vi "Test10.vi"(5 "Peak":T2=enum."PCAN_USBBUS1", 7 "L2T":T1 caption="Limites de test pris en compte", 8 "errin":errorcluster, 9 "SN":string="0B5MEVA000CA1JC1M0000041", 10 "OCV":string) -> (0 "errout":errorcluster, 2 "chaîne concaténée":string, 4 "cluster de sortie":T3, 6 "v1":string)   [LabVIEW 2020]
uses:
  <userlib>/PCAN Basic/Controls/Channel.ctl
  Ctrl/L2T.ctl
  VarGLO/Global var.vi
  <vilib>/regexp/Match Regular Expression.xnode
  <userlib>/PCAN Basic/PCANBasic.lvlib
panel:
  out "String out":string
  # "Pre DCIR_____________________________________"
  # "intra DCIR_____________________________________"
  # "Post DCIR_____________________________________"
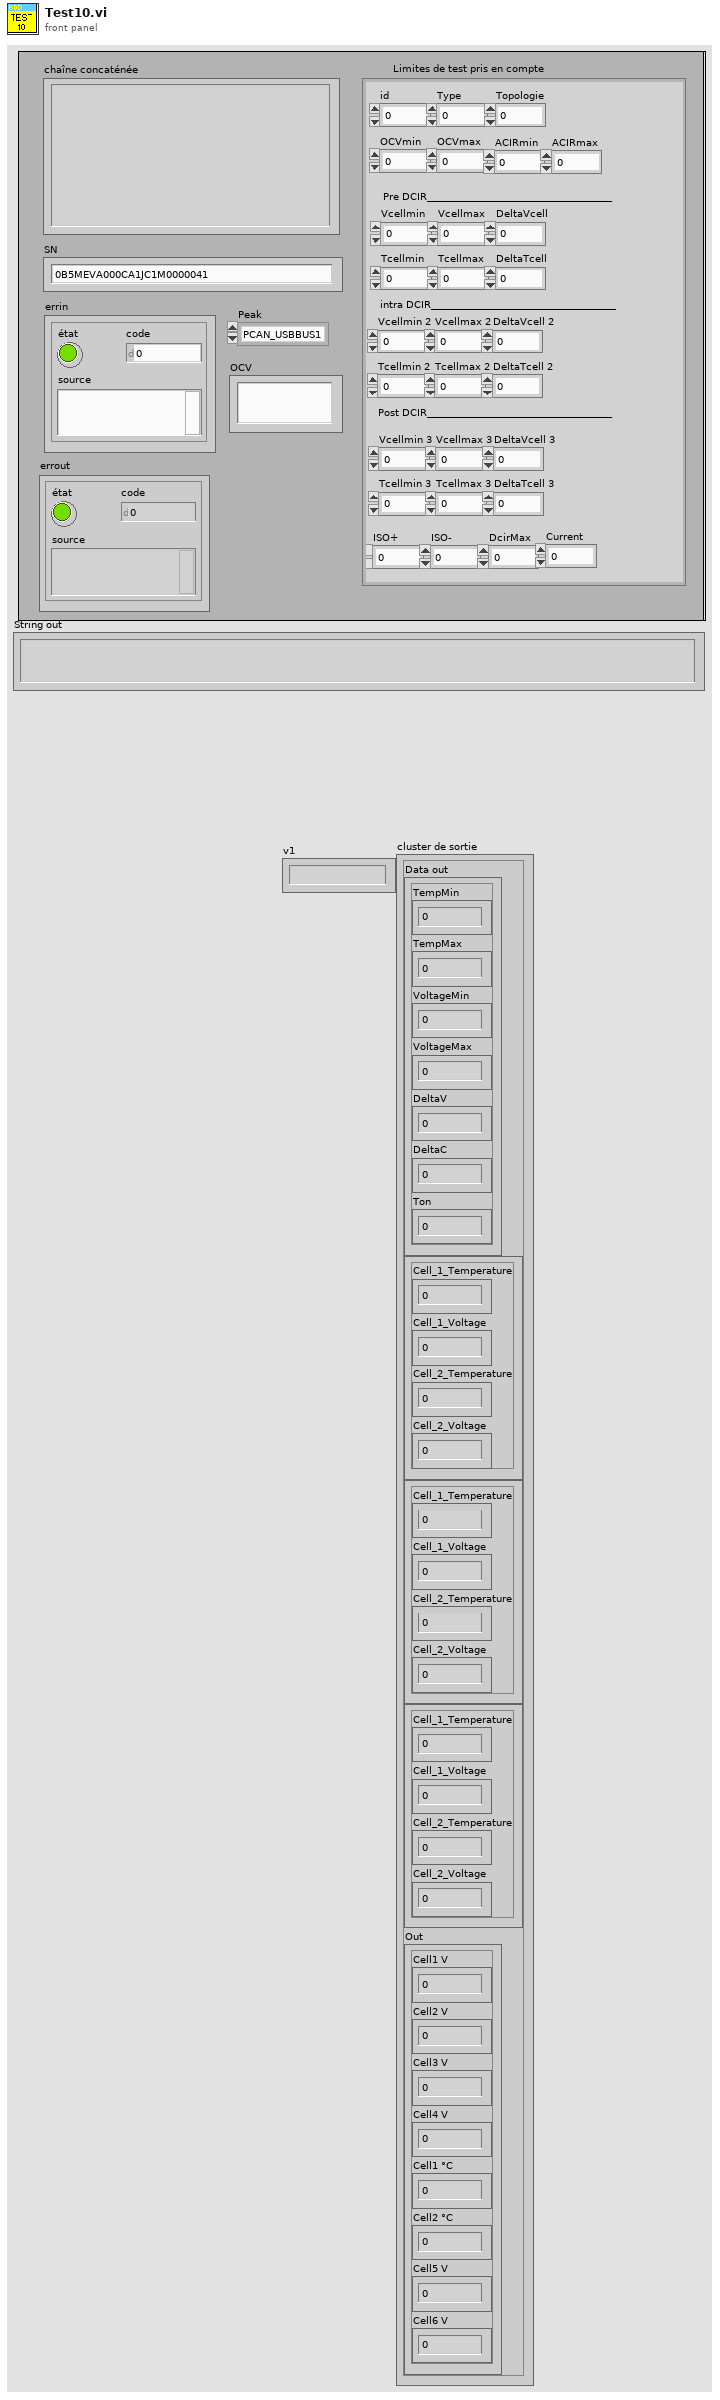
[diagram p1: front panel]
types:
  T1 = typedef "L2T.ctl" = cluster{"id":dbl, "Type":dbl, "OCVmin":dbl, "OCVmax":dbl, "ACIRmin":dbl, "ACIRmax":dbl, "Vcellmin":dbl, "Vcellmax":dbl, "DeltaVcell":dbl, "Tcellmin":dbl, "Tcellmax":dbl, "DeltaTcell":dbl, "ISO+":dbl, "ISO-":dbl, "DcirMax":dbl, "Current":dbl, "Topologie":dbl, "Vcellmin 2":dbl, "Vcellmax 2":dbl, "DeltaVcell 2":dbl, "Tcellmin 2":dbl, "Tcellmax 2":dbl, "DeltaTcell 2":dbl, "Vcellmin 3":dbl, "Vcellmax 3":dbl, "DeltaVcell 3":dbl, "Tcellmin 3":dbl, "Tcellmax 3":dbl, "DeltaTcell 3":dbl}
  T2 = typedef "PCANBasic.lvlib/Channel.ctl" = enum16{"PCAN_NONEBUS", "not used1", "not used2", "not used3", "not used4", "not used5", "not used6", "not used7", "not used8", "not used9", "not used10", "not used11", "not used12", "not used13", "not used14", "not used15", "not used16", "not used17", "not used18", "not used19", "not used20", "not used21", "not used22", "not used23", "not used24", "not used25", "not used26", "not used27", "not used28", "not used29", "not used30", "not used31", "not used32", "PCAN_ISABUS1", "PCAN_ISABUS2", "PCAN_ISABUS3", "PCAN_ISABUS4", "PCAN_ISABUS5", "PCAN_ISABUS6", "PCAN_ISABUS7", "PCAN_ISABUS8", "not used41", "not used42", "not used43", "not used44", "not used45", "not used46", "not used47", "not used48", "PCAN_DNGBUS1", "not used50", "not used51", "not used52", "not used53", "not used54", "not used55", "not used56", "not used57", "not used58", "not used59", "not used60", "not used61", "not used62", "not used63", "not used64", "PCAN_PCIBUS1", "PCAN_PCIBUS2", "PCAN_PCIBUS3", "PCAN_PCIBUS4", "PCAN_PCIBUS5", "PCAN_PCIBUS6", "PCAN_PCIBUS7", "PCAN_PCIBUS8", "not used73", "not used74", "not used75", "not used76", "not used77", "not used78", "not used79", "not used80", "PCAN_USBBUS1", "PCAN_USBBUS2", "PCAN_USBBUS3", "PCAN_USBBUS4", "PCAN_USBBUS5", "PCAN_USBBUS6", "PCAN_USBBUS7", "PCAN_USBBUS8", "Not used89", "Not used90", "Not used91", "Not used92", "Not used93", "Not used94", "Not used95", "Not used96", "PCAN_PCCBUS1", "PCAN_PCCBUS2"}
  T3 = cluster{"Data out":cluster{"TempMin":sgl, "TempMax":sgl, "VoltageMin":sgl, "VoltageMax":sgl, "DeltaV":sgl, "DeltaC":sgl, "Ton":sgl}, "Cluster":cluster{"Cell_1_Temperature":sgl, "Cell_1_Voltage":sgl, "Cell_2_Temperature":sgl, "Cell_2_Voltage":sgl}, "Cluster":cluster{"Cell_1_Temperature":sgl, "Cell_1_Voltage":sgl, "Cell_2_Temperature":sgl, "Cell_2_Voltage":sgl}, "Cluster":cluster{"Cell_1_Temperature":sgl, "Cell_1_Voltage":sgl, "Cell_2_Temperature":sgl, "Cell_2_Voltage":sgl}, "Out":cluster{"Cell1 V":sgl, "Cell2 V":sgl, "Cell3 V":sgl, "Cell4 V":sgl, "Cell1 °C":sgl, "Cell2 °C":sgl, "Cell5 V":sgl, "Cell6 V":sgl}}
  T4 = cluster{"Cell1 V":sgl, "Cell2 V":sgl, "Cell3 V":sgl, "Cell4 V":sgl, "Cell1 °C":sgl, "Cell2 °C":sgl, "Cell5 V":sgl, "Cell6 V":sgl}
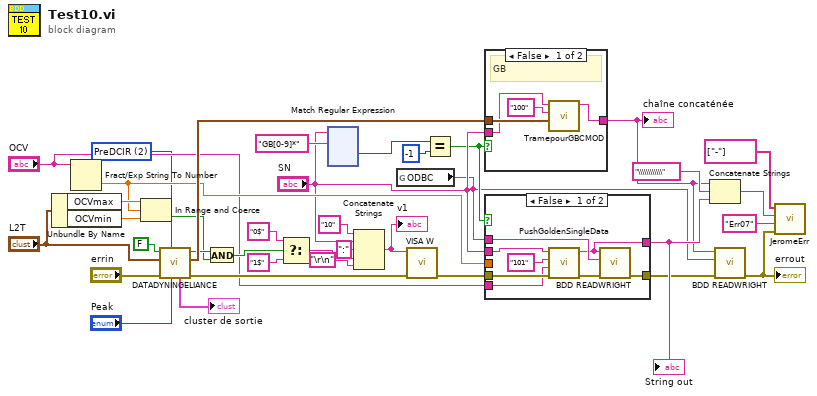
[diagram p0: block diagram]
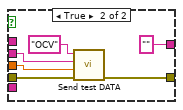
[diagram p2: hidden frame]
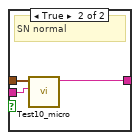
[diagram p3: hidden frame]
diagram:
  w1 = u16 2 items=["PostDCIR", "intraDCIR", "PreDCIR"] ("StepCMOD")
  n1 = Unbundle By Name("L2T") -> ("OCVmax"=w34:dbl, "OCVmin"=w33:dbl)
  n2 = Fract/Exp String To Number ("Chaîne Fract/Exp en nombre")(string="OCV") -> (number=w24:dbl)  [unwired: 3 in, 1 out]
  n3 = In Range and Coerce(upper limit=w34, x=w24, lower limit=w33) -> (In Range?=w29:bool)  [unwired: 1 out]
  n4 = call "DATADYNINGELIANCE.vi"("Channel"="Peak", "StepCMOD"=w1, "errin"="errin", "L2T"="L2T", "3P4S"=FALSE) -> ("errout"=w19:errorcluster, "Out"=w37:T4, "test OK?"=w30:bool, "cluster de sortie"=→"cluster de sortie":T3)  [unwired: 2 in, 1 out]
  n5 = And(x=w30, y=w29) -> (x .and. y?=w28:bool)
  n6 = Select(t="0$" ("chaîne"), s=w28, f="1$" ("chaîne")) -> (s? t:f=w26:string)
  n7 = xnode "Match Regular Expression"("input string"="SN", "regular expression"="GB[0-9]*") -> ("offset past match"=w14:i32)  [unwired: 4 in, 4 out]
  n8 = Concatenate Strings("10" ("chaîne"), "SN", ":" ("string"), w26, "\r\n") -> (w17:string)
  "v1" <- w17
  n9 = global read "Global var.vi" "ODBC"() -> (w8:string)
  n10 = call "VISA W.vi"("errin"=w19, "Chaîne"=w17) -> ("errout"=w18:errorcluster)  [unwired: 9 in]
  n11 = Equal?(x=w14, y=-1) -> (x = y?=w11:bool)
  n12 = case shown="False" w11 {
    tunnel: w37 -> [w41 w44]
    tunnel: [w40 w43] -> w5
    tunnel: "SN" -> [w39 w42]
    frame False {
      # "GB"
      n13 = call "TramepourGBCMOD.vi"("Out"=w41, "TestNum"="100", "SN"=w39) -> ("String"=w40:string)  [unwired: 8 in]
    }
    frame True {
      # "SN normal"
      n14 = call "Test10_micro.vi"("SN"=w42, "Out"=w44) -> ("String"=w43:string)  [unwired: 9 in]
    }
  }
  "chaîne concaténée" <- w5
  n15 = case shown="False" w11 {
    tunnel: w24 -> [_ w57]
    tunnel: w18 -> [w51 w56]
    tunnel: [w48 w55] -> w7
    tunnel: "SN" -> [w52 w54]
    tunnel: [w46 "" ("String out")] -> w9
    tunnel: w8 -> [w47 _]
    tunnel: "OCV" -> [w45 _]
    frame False {
      n16 = call "PushGoldenSingleData.vi"("errin"=w51, "Value"=w45, "TestNum"="101", "SN"=w52) -> ("errout"=w49:errorcluster, "String out"=w46:string)  [unwired: 6 in]
      n17 = call <userlib>:"BDD READWRIGHT.vi"("errin"=w49, "DSN name"=w47, "Instruction"=w46) -> ("error out"=w48:errorcluster)  [unwired: 7 in, 1 out]
    }
    frame True {
      n18 = call "Send test DATA.vi"("errin"=w56, "Value"=w57, "SN"=w54, "test"="OCV") -> ("error out"=w55:errorcluster)  [unwired: 7 in]
    }
  }
  "String out" <- w9
  n19 = Concatenate Strings(w5, "\\\\\\\\\\\\" ("string"), w9) -> (w4:string)
  n20 = call <userlib>:"BDD READWRIGHT.vi"("errin"=w7, "DSN name"=w8, "Instruction"=w5) -> ("error out"=w6:errorcluster)  [unwired: 7 in, 1 out]
  "errout" <- w6
  n21 = call "JeromeErr.vi"("Errin"=w6, "CodeERR"="Err07", "RequetteSQL"=w4, "RetourSQL"=string[] ["-"]) -> ()  [unwired: 8 in]
